vi "Write Yield Counts.vi"(8 "error in (no error)":errorcluster, 10 "DatasFiles.DataWrite":variant, 11 "Master in":refnum<class "Master.lvclass">) -> (0 "error out":errorcluster, 3 "Master out":refnum<class "Master.lvclass">)   [LabVIEW 2014, in "Master.lvclass"]
uses:
  Master/Master.lvclass
  Master/Master.lvclass/Master.ctl
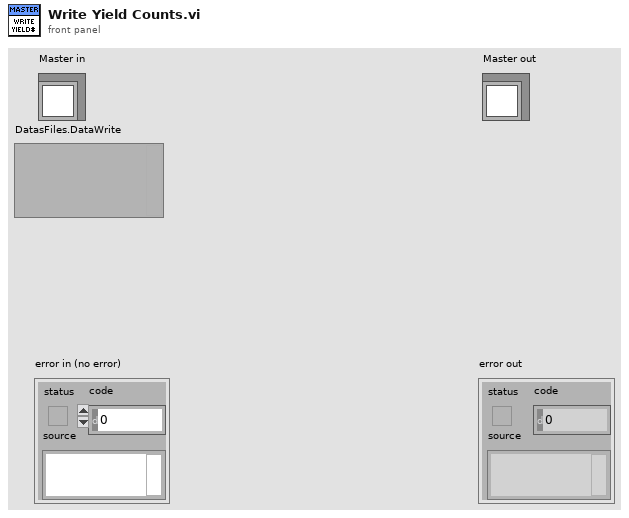
[diagram p1: front panel]
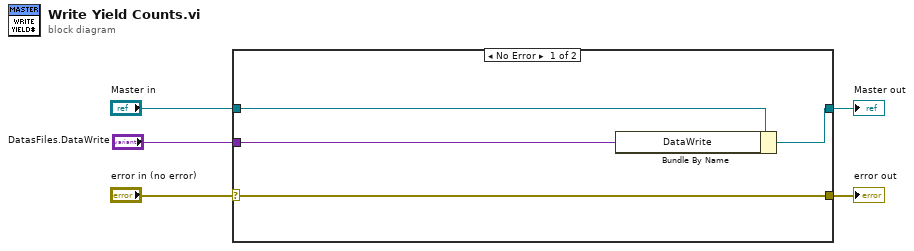
[diagram p0: block diagram]
diagram:
  n1 = case shown="No Error" "error in (no error)" {
    selector: "error in (no error)" -> [w9 w11]
    tunnel: [w9 w11] -> w4
    tunnel: [w7 w10] -> w2
    tunnel: "Master in" -> [w8 w10]
    tunnel: "DatasFiles.DataWrite" -> [w6 _]
    frame No Error {
      n2 = Bundle By Name(cluster=w8, "DataWrite"=w6) -> (w7:refnum<class "Master.lvclass">)
    }
    frame Error {
    }
  }
  "error out" <- w4
  "Master out" <- w2
